vi "通讯全局变量断电保存.vi"() -> ()   [LabVIEW 2016, in "采配水.lvlib"]
panel:
  in  "运行周期":T1={"运行模式"=enum."维护模式", "质控频次"=enum."关闭", "空白核查时间"=2, "跨度核查时间"=6, "24H周期设置"=[]} {"跨度核查时间" items=["00H", "01H", "02H", "03H", "04H", "05H", "06H", "07H", "08H", "09H", "10H", "11H", "12H", "13H", "14H", "15H", "16H", "17H", "18H", "19H", "20H", "21H", "22H", "23H", "关闭"]; "空白核查时间" items=["00H", "01H", "02H", "03H", "04H", "05H", "06H", "07H", "08H", "09H", "10H", "11H", "12H", "13H", "14H", "15H", "16H", "17H", "18H", "19H", "20H", "21H", "22H", "23H", "关闭"]}
  in  "自动补水":bool=TRUE
  in  "排气扇参数":T2={"功能开关"=enum."关闭", "排气扇开启温度"=50.0, "排气扇关闭温度"=40.0}
  in  "冰箱参数":T3={"功能开关"=enum."关闭", "开启时间"=6, "关闭时间"=20} {"关闭时间" items=["00H", "01H", "02H", "03H", "04H", "05H", "06H", "07H", "08H", "09H", "10H", "11H", "12H", "13H", "14H", "15H", "16H", "17H", "18H", "19H", "20H", "21H", "22H", "23H", "关闭"]; "开启时间" items=["00H", "01H", "02H", "03H", "04H", "05H", "06H", "07H", "08H", "09H", "10H", "11H", "12H", "13H", "14H", "15H", "16H", "17H", "18H", "19H", "20H", "21H", "22H", "23H", "关闭"]}
  in  "采配水参数":T4={"排空时间"=60.0, "润洗时间"=60.0, "进样超时时间"=300.0, "沉淀时间"=1800.0, "配水时间"=7200.0}
  in  "ZLAN 启用":bool=TRUE
  in  "ZLAN IP":string="192.168.1.200"
  in  "报警参数配置":T5={"低压报警阈值 V"=22.0, "低压报警解除阈值 V"=25.0, "高温报警阈值 ℃"=50.0, "高温报警解除阈值 ℃"=40.0, "湿度报警阈值 %"=95.0, "湿度报警解除阈值 %"=90.0}
  # "运行模式："
  # "质控频次："
  # "零点核查时间："
  # "跨度核查时间："
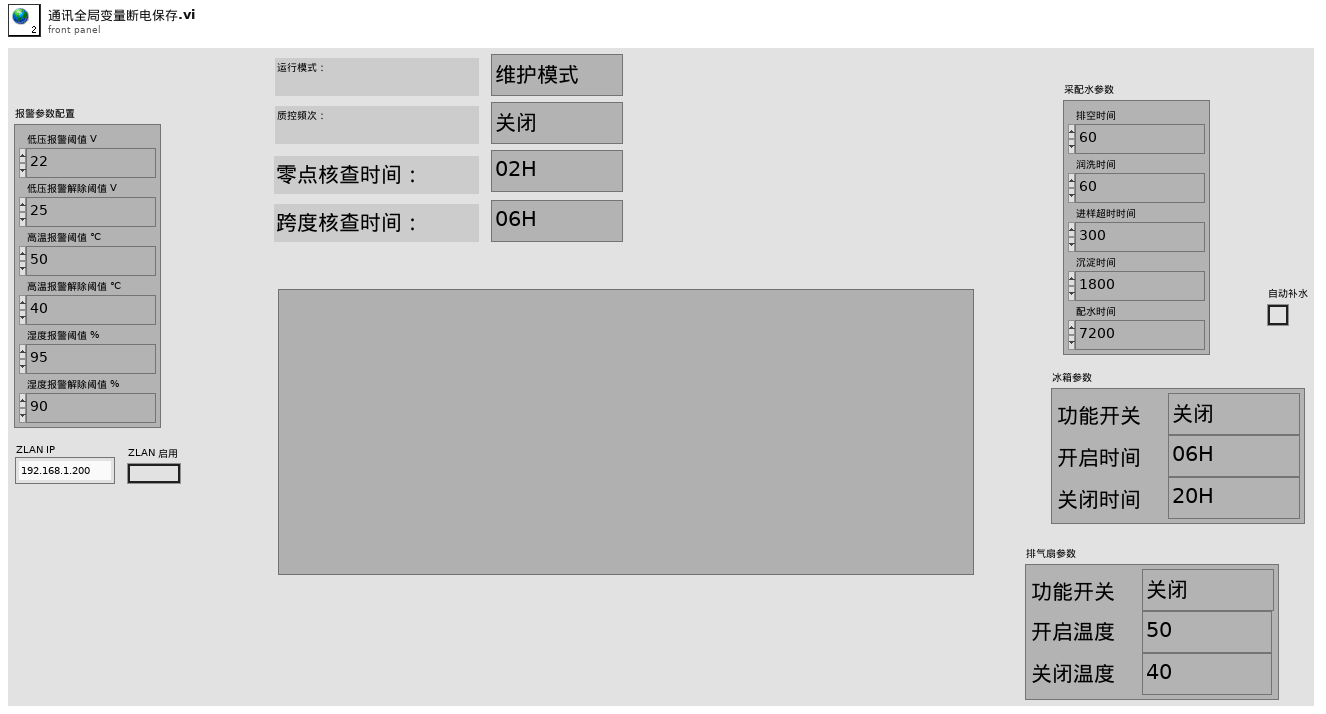
[diagram p1: front panel]
types:
  T1 = cluster{"运行模式":enum16{"维护模式", "常规模式", "应急模式", "质控模式"}, "质控频次":enum16{"关闭", "每天", "星期一", "星期二", "星期三", "星期四", "星期五", "星期六", "星期日"}, "空白核查时间":u16, "跨度核查时间":u16, "24H周期设置":bool[]}
  T2 = cluster{"功能开关":enum16{"关闭", "开启"}, "排气扇开启温度":dbl, "排气扇关闭温度":dbl}
  T3 = cluster{"功能开关":enum16{"关闭", "开启"}, "开启时间":u16, "关闭时间":u16}
  T4 = cluster{"排空时间":dbl, "润洗时间":dbl, "进样超时时间":dbl, "沉淀时间":dbl, "配水时间":dbl}
  T5 = cluster{"低压报警阈值 V":dbl, "低压报警解除阈值 V":dbl, "高温报警阈值 ℃":dbl, "高温报警解除阈值 ℃":dbl, "湿度报警阈值 %":dbl, "湿度报警解除阈值 %":dbl}
diagram:
